vi "Extract Message.vi"(6 "Paras In":variant, 8 "error in (no error)":errorcluster, 9 "Priority":i32, 10 "Wait":i32=-1, 11 "System Actor in":refnum<class "System Actor.lvclass">) -> (0 "error out":errorcluster, 1 "Valid":bool, 2 "Message Out":refnum<class "Message.lvclass">, 3 "System Actor out":refnum<class "System Actor.lvclass">)   [LabVIEW 2024, in "System Actor.lvclass"]
uses:
  System Actor.lvclass
  Message/Message.lvclass
  System Actor.lvclass/System Actor.ctl
  Public Data/Call Messenger.vi
  Messenger/Messenger/Messenger.lvclass
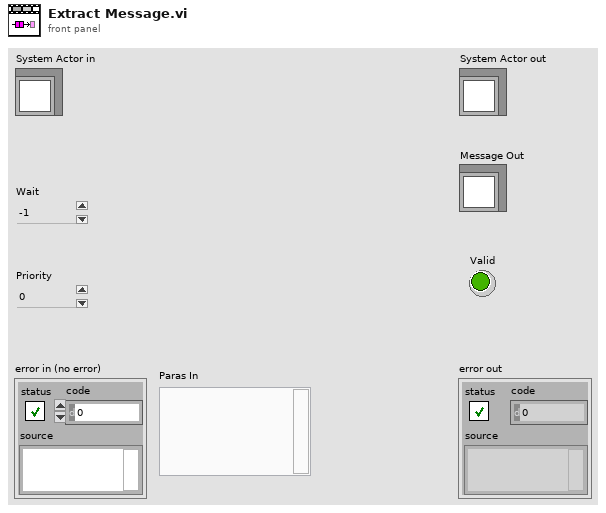
[diagram p1: front panel]
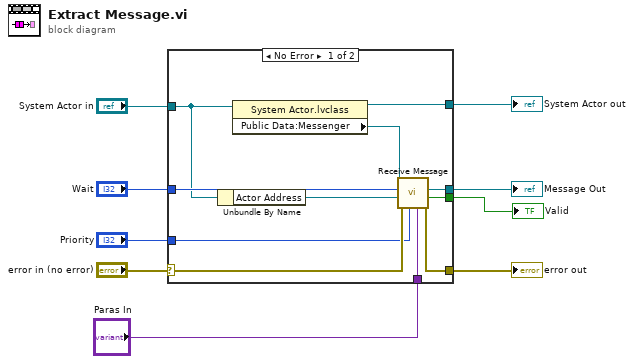
[diagram p0: block diagram]
diagram:
  n1 = case shown="No Error" "error in (no error)" {
    selector: "error in (no error)" -> [w18 w22]
    tunnel: [w17 w22] -> w8
    tunnel: [w13 w21] -> w6
    tunnel: "System Actor in" -> [w15 w21]
    tunnel: [w20 _] -> w5
    tunnel: [w19 _] -> w4
    tunnel: "Wait" -> [w16 _]
    tunnel: "Priority" -> [w11 _]
    tunnel: "Paras In" -> [w10 _]
    frame No Error {
      n2 = Unbundle By Name(w15) -> ("Actor Address"=w12:refnum<class "Mail Strategy.lvclass">)
      n3 = property class="System Actor.lvclass"(reference=w15) -> (reference out=w13:refnum<class "System Actor.lvclass">, "Public Data:Messenger"=w14:refnum<class "Messenger.lvclass">)  [unwired: 1 in, 1 out]
      n4 = call-dynamic "Receive Message.vi"("Paras In"=w10, "Priority"=w11, "error in (no error)"=w18, "Mail Strategy In"=w12, "Wait(ms)"=w16, "Messenger Component in"=w14) -> ("error out"=w17:errorcluster, "Valid"=w19:bool, "Message Out"=w20:refnum<class "Message.lvclass">)  [unwired: 2 in, 1 out]
    }
    frame Error {
    }
  }
  "error out" <- w8
  "System Actor out" <- w6
  "Message Out" <- w5
  "Valid" <- w4
